vi "PowerIn MSMT Get ET Timing Step from DB.vi"(8 "error in (no error)":errorcluster, 11 "Servo MSMT in":refnum<class "Input Power Measurement.lvclass">) -> (0 "error out":errorcluster, 2 "Step Out":refnum<k7>, 3 "Servo MSMT out":refnum<class "Input Power Measurement.lvclass">)   [LabVIEW 2014, in "Input Power Measurement.lvclass"]
uses:
  Input Power Measurement.lvclass
  QPA Measurement/QPA Measurement.lvlibp/Sequence Automation/Classes/QPA Measurement/Protected Methods/Read Measurement Name.vi
  QPA Measurement/QPA Measurement.lvlibp/Sequence Automation/Classes/QPA Measurement/QPA Measurement.lvclass
  TestStand API Tools/Step Actions/TSAT Step Actions.lvlib
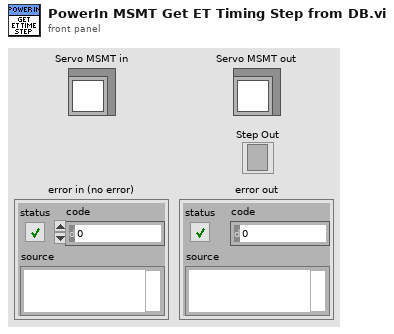
[diagram p1: front panel]
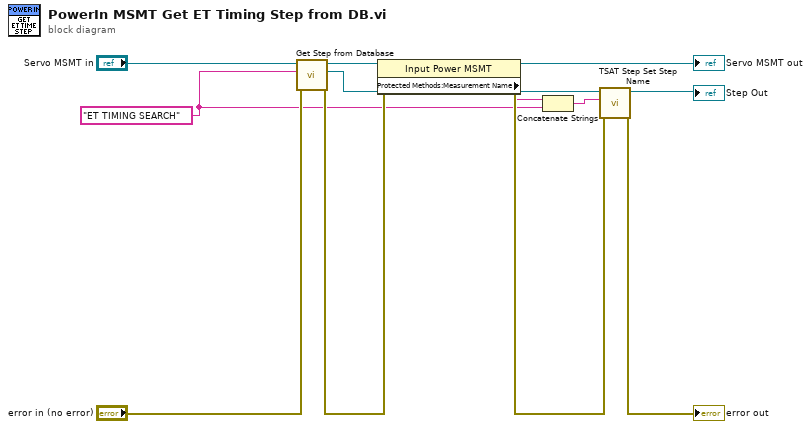
[diagram p0: block diagram]
diagram:
  w1 = "ET TIMING SEARCH" ("string")
  n1 = call "Get Step from Database.vi"("error in (no error)"="error in (no error)", "Default Step"=w1, "QPA Measurement in"="Servo MSMT in") -> ("error out"=w7:errorcluster, "Step Out"=w10:refnum<k7>, "QPA Measurement out"=w5:refnum<class "Input Power Measurement.lvclass">)  [unwired: 6 in]
  n2 = property class="Input Power MSMT"(reference=w5, error in=w7) -> (reference out=→"Servo MSMT out":refnum<class "Input Power Measurement.lvclass">, error out=w6:errorcluster, "Protected Methods:Measurement Name"=w3:string)
  n3 = Concatenate Strings(w3, w1) -> (w2:string)
  n4 = call "TSAT Step Set Step Name.vi"("Error In"=w6, "Name"=w2, "Step In"=w10) -> ("Error Out"=→"error out":errorcluster, "Step Out"=→"Step Out":refnum<k7>)  [unwired: 7 in]
